vi "Launch.vi"(5 "Status Q":refnum<class "MessageQ.lvclass">, 7 "VolatusAPI":refnum<class "VolatusAPI.lvclass">, 8 "error in (no error)":errorcluster, 9 "Config":refnum<class "VolatusConfigElement.lvclass">) -> (0 "error out":errorcluster, 2 "MessageQ":refnum<class "MessageQ.lvclass">)   [LabVIEW 2020, in "Volatus.lvlib" / "Event Reporter Module.lvclass"]
uses:
  Event Reporter Module.lvclass
  MessageQ/MessageQ.lvclass
  VolatusAPI/VolatusAPI.lvclass
  VolatusConfig/VolatusConfigElement/VolatusConfigElement.lvclass
  C:/dev/lv20CE/relink/lv-volatus/Volatus/Module/Module.lvclass
  Event Reporter Module.lvclass/Event Reporter Module.ctl
  lv-exec-anchor/ExecAnchor/ExecAnchor.lvclass
  Module/Module.lvclass
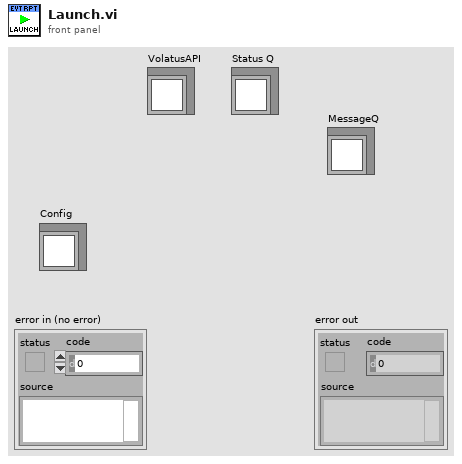
[diagram p1: front panel]
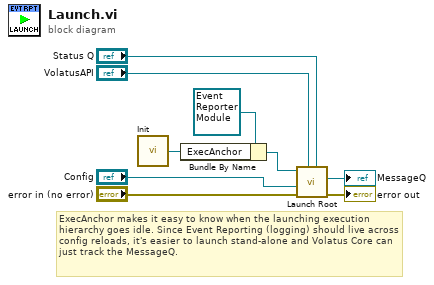
[diagram p0: block diagram]
diagram:
  # "ExecAnchor makes it easy to know when the launching execution hierarchy goes idle. Since Event Reporting (logging) should live across config reloads, it's easier to launch stand-alone and Volatus Core can just track the MessageQ."
  n1 = call "Init.vi"() -> ("ExecAnchor out"=w8:refnum<class "ExecAnchor.lvclass">)  [unwired: 7 in]
  n2 = Bundle By Name(cluster=refnum<class "Event Reporter Module.lvclass"> refnum ("Event Reporter Module in"), "ExecAnchor"=w8) -> (w7:refnum<class "Event Reporter Module.lvclass">)
  n3 = call "Launch Root.vi"("Status Q"="Status Q", "VolatusAPI"="VolatusAPI", "error in (no error)"="error in (no error)", "Config Element"="Config", "Module in"=w7) -> ("error out"=→"error out":errorcluster, "MessageQ"=→"MessageQ":refnum<class "MessageQ.lvclass">)  [unwired: 5 in]
